vi "_Hololens_GaitDisplay.vi"() -> ()   [LabVIEW 2016]
uses:
  <vilib>/HaroTek/Haro3D/Utilities/3D objects/3D_Shape_class/3D_Shape.lvclass
  Classes/CAlex2-Display/CAlex2_Display.lvclass
  C:/Users/Rand/Documents/CAlex2-controller/Classes/CAlex2/CAlex2.lvclass
  C:/Users/Rand/Documents/CAlex2-controller/Classes/SerialChain/SerialChain.lvclass
  Classes/CAlex2/TypeDef/LowerBodyDim.ctl
  Classes/CAlex2/CAlex2.lvclass
  Classes/SerialChain/SerialChain.lvclass
  <vilib>/HaroTek/Haro3D/Hololens/Hololens_class/Hololens.lvclass
panel:
  in  "Shape":refnum<class "3D_Shape.lvclass">
  in  "XY":bool
  in  "Leg Position":refnum<k7>(container)
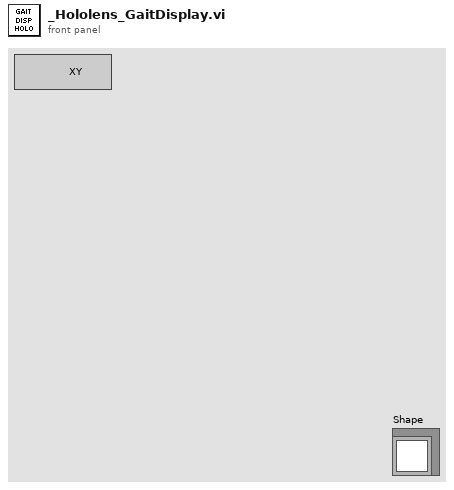
[diagram p1: front panel]
types:
  T1 = enum32{"Invalid", "Standard", "Closed", "Hidden", "Minimized", "Maximized"}
  T2 = cluster{"AxisLabel":string[], "AxisMax":dbl[], "AxisMin":dbl[]}
  T3 = typedef "CAlex2.lvclass/LowerBodyDim.ctl" = cluster{"BodyDim":cluster{"ThighLt (m)":dbl, "ShankLt (m)":dbl, "HipWd (m)":dbl}, "BodyWt":cluster{"Thigh (kg)":dbl, "Shank (kg)":dbl}, "Cuff Loc":cluster{"HipCuffWd (m)":dbl, "HipCuffHt (m)":dbl, "HipFwdShift (m)":dbl, "ThighToKnee (m)":dbl, "ThighCuffDist (m)":dbl, "ShankToKnee (m)":dbl}}
  T4 = typedef "imagedata.ctl" = cluster{"image type":i32, "image depth":i32, "image":u8[], "mask":u8[], "colors":u32[], "Rectangle":cluster{"left":i16, "top":i16, "right":i16, "bottom":i16}}
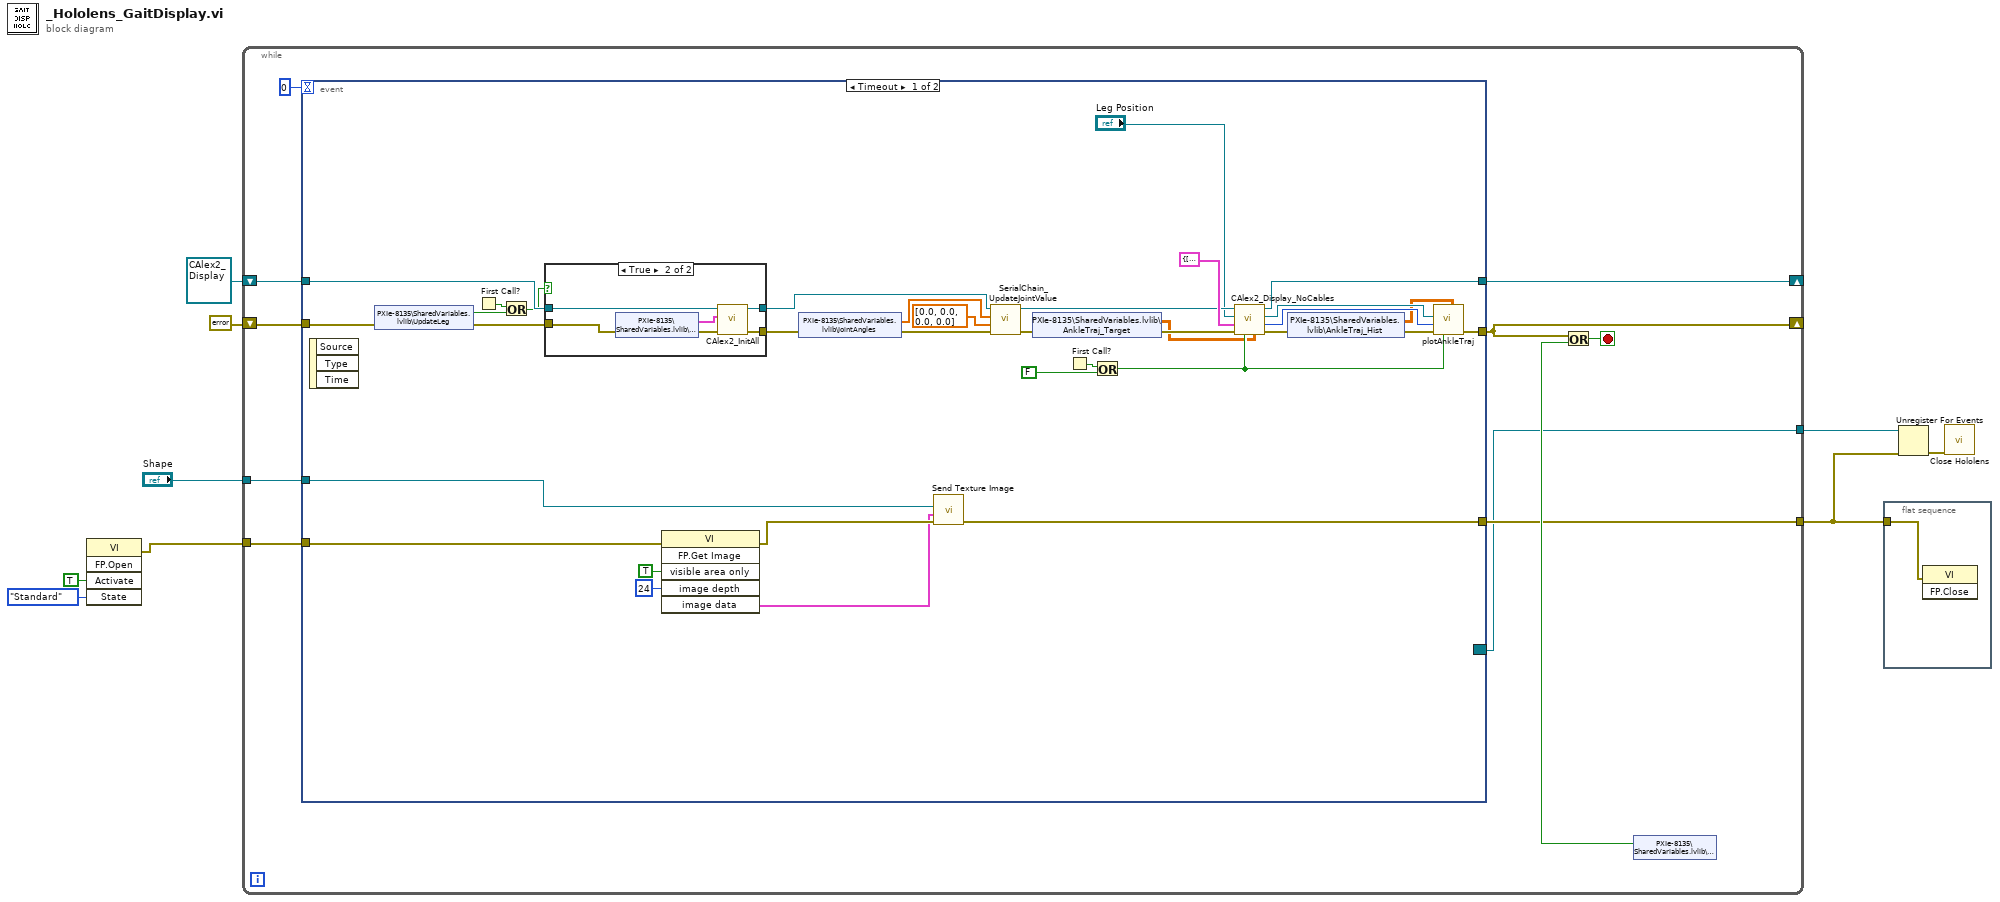
[diagram p0: block diagram]
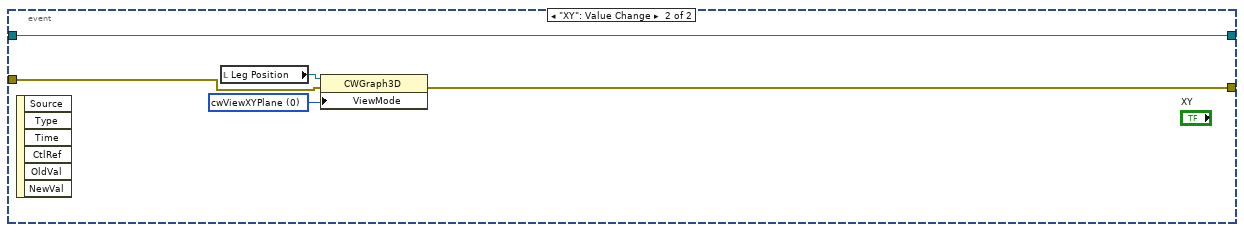
[diagram p3: hidden frame]
diagram:
  n1 = invoke class="VI" method="FP.Open"("Activate"=TRUE ("Activate?"), "State"=T1."Standard") -> (error out=w5:errorcluster)  [unwired: 3 in, 4 out]
  n2 = while {
    shift-right: [w18] -> _
    shift-left: refnum<class "CAlex2_Display.lvclass"> refnum ("CAlex2") -> [w19]
    shift-right: [w17] -> _
    shift-left: errorcluster {"status"=FALSE, "code"=0, "source"=""} ("error out") -> [w14]
    tunnel: w5 -> [w13]
    tunnel: [w12] -> w4
    tunnel: [w11] -> w2
    tunnel: "Shape" -> [w10]
    stop <- w15 stop-if-true
    n3 = event shown="[0] Timeout" {
      selector: _ -> [_ _]
      dyn-events: [_ _] -> w11
      timeout: 0 -> [_ _]
      tunnel: w19 -> [w43 w63]
      tunnel: [w45 w63] -> w18
      tunnel: [w44 w65] -> w17
      tunnel: w14 -> [w40 w66]
      tunnel: w13 -> [w25 _]
      tunnel: [w23 _] -> w12
      tunnel: w10 -> [w21 _]
      event Timeout {
        n4 = event-data() -> ()  [unwired: 1 in, 3 out]
        n5 = shared-variable "PXIe-8135\\SharedVariables.lvlib\\UpdateLeg"(error in=w40) -> (w36:bool, error out=w39:errorcluster)
        n6 = First Call?() -> (First Call?: T/F=w37:bool)
        n7 = Or(x=w37, y=w36) -> (x .or. y?=w35:bool)
        n8 = case shown="True" w35 {
          tunnel: w43 -> [w56 w62]
          tunnel: [w56 w61] -> w42
          tunnel: [w55 w58] -> w41
          tunnel: w39 -> [w55 w57]
          frame False {
          }
          frame True {
            n9 = shared-variable "PXIe-8135\\SharedVariables.lvlib\\LegDim"(error in=w57) -> (w60:T3, error out=w59:errorcluster)
            n10 = call "CAlex2_InitAll.vi"("error in (no error)"=w59, "LegProperties"=w60, "CAlex2 in"=w62) -> ("error out"=w58:errorcluster, "CAlex2 out"=w61:refnum<class "CAlex2_Display.lvclass">)  [unwired: 7 in]
          }
        }
        n11 = invoke class="VI" method="FP.Get Image"(error in=w25, "visible area only"=TRUE ("Visible Area Only"), "image depth"=24 ("Image Depth")) -> (error out=w24:errorcluster, "image data"=w22:T4)  [unwired: 3 in, 4 out]
        n12 = shared-variable "PXIe-8135\\SharedVariables.lvlib\\JointAngles"(error in=w41) -> (w53:dbl[], error out=w52:errorcluster)
        n13 = call <vilib>:"Send Texture Image.vi"("error in (no error)"=w24, "Texture (no texture)"=w22, "Shape"=w21) -> ("error out"=w23:errorcluster)  [unwired: 8 in]
        n14 = call "SerialChain_UpdateJointValue.vi"("error in (no error)"=w52, "JointSpeed (rad/s | m/s)"=dbl[] [0.0, 0.0, 0.0, 0.0] ("JointSpeed (rad)"), "JointAngle (rad | m)"=w53, "SerialChain in"=w42) -> ("error out"=w29:errorcluster, "SerialChain out"=w46:refnum<class "CAlex2_Display.lvclass">)  [unwired: 6 in]
        n15 = shared-variable "PXIe-8135\\SharedVariables.lvlib\\AnkleTraj_Target"(error in=w29) -> (w28:dbl[][], error out=w30:errorcluster)
        n16 = First Call?() -> (First Call?: T/F=w51:bool)
        n17 = Or(x=w51, y=FALSE ("Reset")) -> (x .or. y?=w47:bool)
        n18 = call "CAlex2_Display_NoCables.vi"("AnkleTraj"=w28, "Init?"=w47, "error in (no error)"=w30, "AxisSetting"=T2 {"AxisLabel"=["x ", "y", "z "], "AxisMax"=[0.75, 0.3, 0.8], "AxisMin"=[-0.75, -1.2, -0.7]}, "3D graph in"="Leg Position", "CLX2 in"=w46) -> ("error out"=w33:errorcluster, "LastPlotNum"=w48:i32, "3D graph out"=w49:refnum<k7>, "CLX2 out"=w45:refnum<class "CAlex2_Display.lvclass">)  [unwired: 2 in]
        n19 = shared-variable "PXIe-8135\\SharedVariables.lvlib\\AnkleTraj_Hist"(error in=w33) -> (w34:dbl[][], error out=w32:errorcluster)
        n20 = call "plotAnkleTraj.vi"("AnkleTraj_history"=w34, "Init?"=w47, "error in (no error)"=w32, "PreviousPlotNum"=w48, "3D graph in"=w49) -> ("error out"=w44:errorcluster)  [unwired: 4 in, 2 out]
      }
      event "XY": Value Change {
        w67 = 0 items=["cwViewXYPlane", "cwViewXZPlane", "cwViewYZPlane", "cwViewUserDefined"] ("ViewMode")
        n21 = event-data() -> ()  [unwired: 1 in, 6 out]
        n22 = local read "Leg Position"() -> (w64:refnum<k7>)
        n23 = property class="CWGraph3D"(reference=w64, error in=w66, "ViewMode"=w67) -> (error out=w65:errorcluster)  [unwired: 1 out]
      }
    }
    n24 = shared-variable "PXIe-8135\\SharedVariables.lvlib\\Stop RT"() -> (w16:bool)  [unwired: 1 in, 1 out]
    n25 = Or(x=w17, y=w16) -> (x .or. y?=w15:bool)
  }
  n26 = flat-sequence {
    tunnel: w4 -> [w68]
    frame #0 {
      n27 = invoke class="VI" method="FP.Close"(error in=w68) -> ()  [unwired: 2 in, 3 out]
    }
  }
  n28 = Unregister For Events(event registration refnum=w2, error in=w4) -> (error out=w3:errorcluster)
  n29 = call <vilib>:"Close Hololens.vi"("error in (no error)"=w3) -> ()  [unwired: 10 in, 1 out]
